vi "Main.vi"(11 "Module Admin":refnum<class "Delacor_lib_QMH_Module Admin.lvclass">) -> ()   [LabVIEW 2020, in "Interface Change.lvlib"]
doc: "This template is based off of the Queued Message Handler design pattern and the Queued Message Handler project template that ships with LabVIEW.\n\nThe main difference is that the queue is private to this module and communication between modules is performed via Broadcast and Request events.\n\nRequest events are wrapped in public API methods and are handled in the Event Handling Loop (EHL) of this VI. Any module can register for Broadcast events sent by this module. The EHL generates messages based on user interface actions.\n\nThe Message Handling Loop (MHL) processes messages generated by the EHL, or by other messages. The messages are string values, so new messages can be added easily to the Message Cases case structure in the MHL. Each message cluster can also provide an optional value for Message Data, which is a variant that can be converted to whatever message-specific data is required.\n_____\nBased on DQMH Project Template 6.1.0.94."
uses:
  Interface Change.lvlib
  <vilib>/Delacor/Delacor QMH/Libraries/Module Admin_class/Delacor_lib_QMH_Module Admin.lvclass
  Module Data--cluster.ctl
  <vilib>/Delacor/Delacor QMH/Libraries/Message Queue_class/Delacor_lib_QMH_Message Queue.lvclass/Delacor_lib_QMH_Message Queue.ctl
  Stop Argument--cluster.ctl
  <vilib>/Delacor/Delacor QMH/Libraries/Module Admin_class/Delacor_lib_QMH_Module Admin.lvclass/Delacor_lib_QMH_Module Admin.ctl
  Change ColorBox Argument--cluster.ctl
  <vilib>/Utility/miscctls.llb/LVPointTypeDef.ctl
  <vilib>/Delacor/Delacor QMH/Libraries/Message Queue_class/Delacor_lib_QMH_Enqueue Message (Single).vi
  <vilib>/Delacor/Delacor QMH/Libraries/Module Admin_class/Delacor_lib_QMH_Get External Launch.vi
  <vilib>/Utility/error.llb/Error Cluster From Error Code.vi
  <vilib>/ErrorRing/Error Ring.xnode
  <vilib>/Delacor/Delacor QMH/Libraries/Message Queue_class/Delacor_lib_QMH_Message Queue.lvclass
panel:
  out "error out":errorcluster
  in  "Simulate MHL Error":bool
  in  "Simulate EHL Error":bool
  # "Other QMH Modules communicate with this Module via its Public API (wrappers for its Request Events).\n\nThis Module communicates with other Modules via its Broadcast Events.\nAny module that wants to get these messages, just registers for this module's Broadcast events."
  # "This template is for the Delacor Modified Queued Message Handler design pattern.\n\nSee the block diagram for more information on how to use this template."
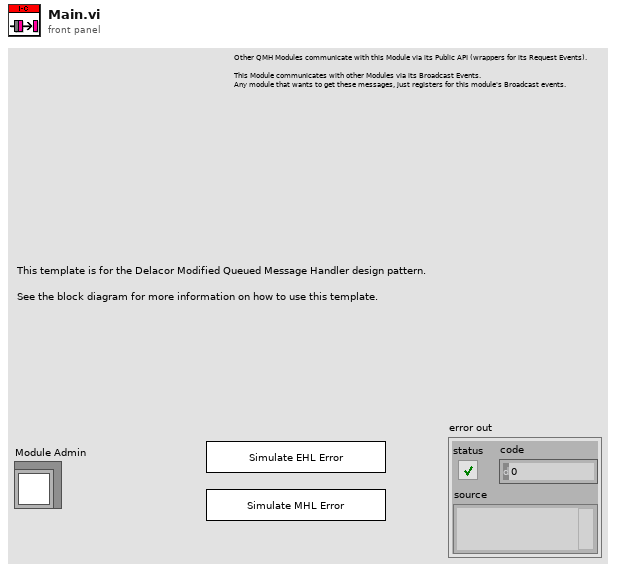
[diagram p1: front panel]
types:
  T1 = typedef "Interface Change.lvlib/Request Events--cluster.ctl" = cluster{"Stop Module":refnum<user-event>, "Show Panel":refnum<user-event>, "Hide Panel":refnum<user-event>, "Get Module Execution Status":refnum<user-event>, "Show Diagram":refnum<user-event>, "Change ColorBox":refnum<user-event>}
  T2 = typedef "Interface Change.lvlib/Module Data--cluster.ctl" = cluster{"Status":string}
  T3 = enum32{"invalid lock state", "Not Locked", "Locked (No Password)", "Password-protected"}
  T4 = typedef "Interface Change.lvlib/Stop Argument--cluster.ctl" = cluster{"Origin":string, "Exit via Stop Module Req?":bool, "Wait for Module to stop?":bool}
  T5 = typedef "Interface Change.lvlib/Change ColorBox Argument--cluster.ctl" = cluster{"Color Box":u32}
  T6 = typedef "LVPointTypeDef.ctl" = cluster{"Horizontal":i16, "Vertical":i16}
  T7 = enum32{"Invalid", "Standard", "Closed", "Hidden", "Minimized", "Maximized"}
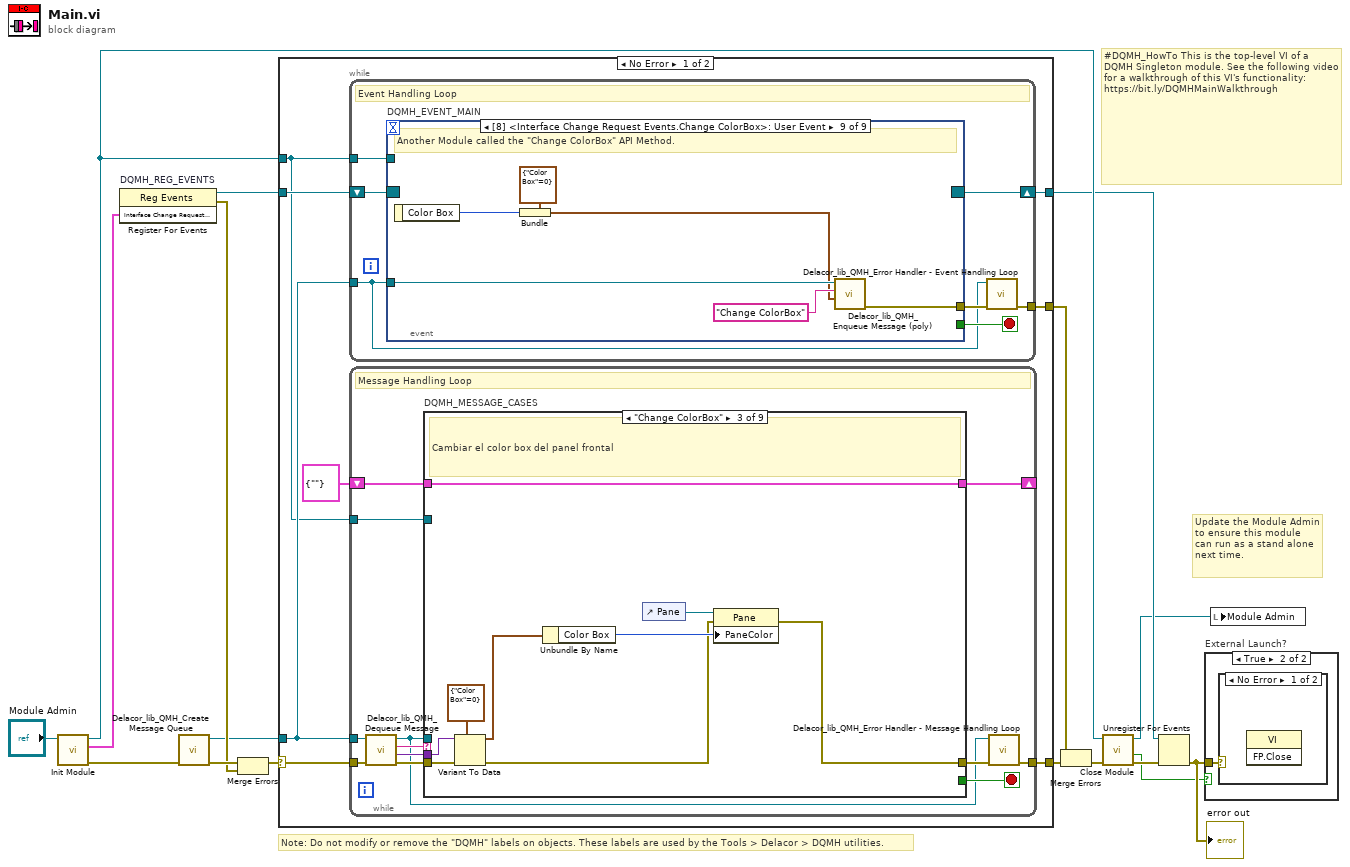
[diagram p0: block diagram]
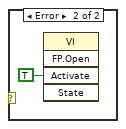
[diagram p3: hidden frame]
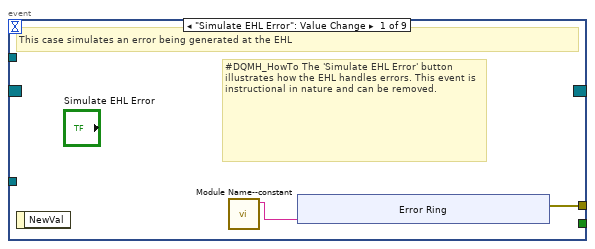
[diagram p4: hidden frame]
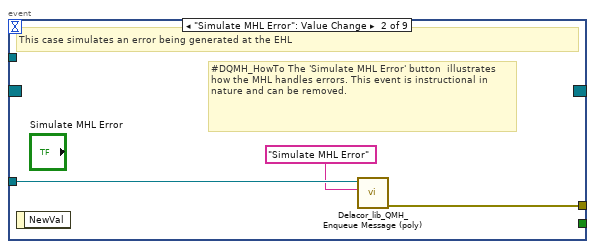
[diagram p5: hidden frame]
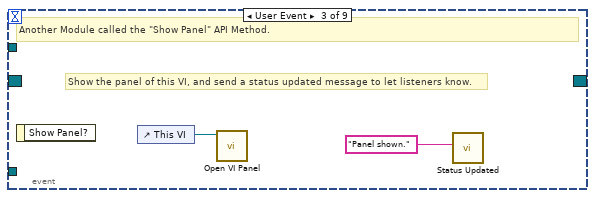
[diagram p6: hidden frame]
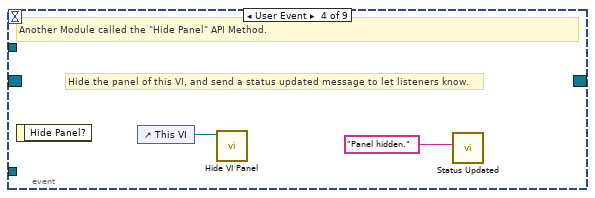
[diagram p7: hidden frame]
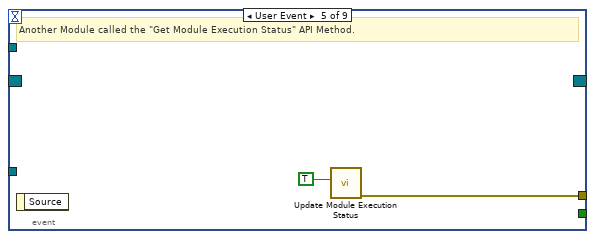
[diagram p8: hidden frame]
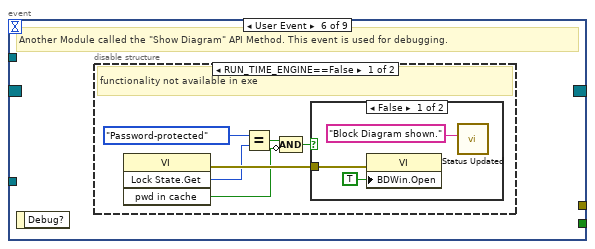
[diagram p9: hidden frame]
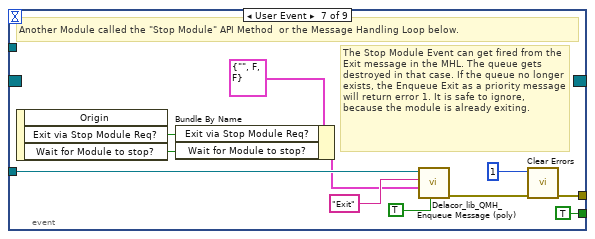
[diagram p12: hidden frame]
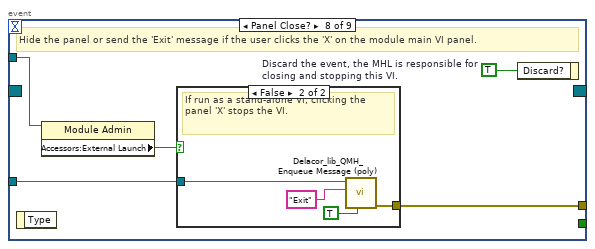
[diagram p13: hidden frame]
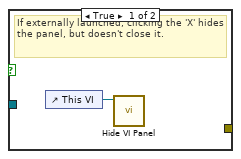
[diagram p14: hidden frame]
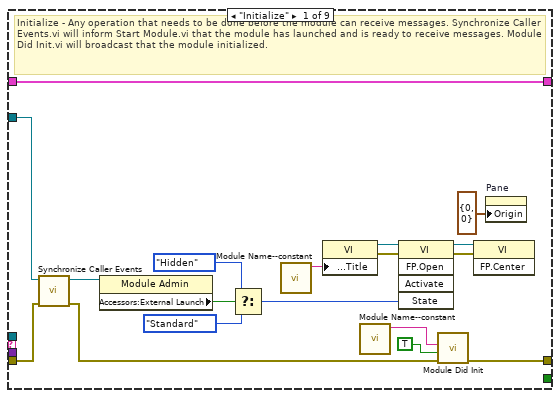
[diagram p15: hidden frame]
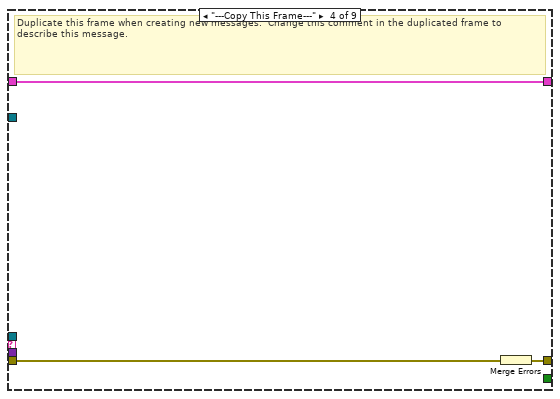
[diagram p17: hidden frame]
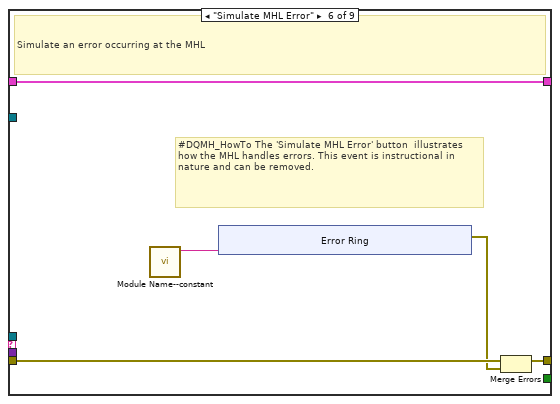
[diagram p19: hidden frame]
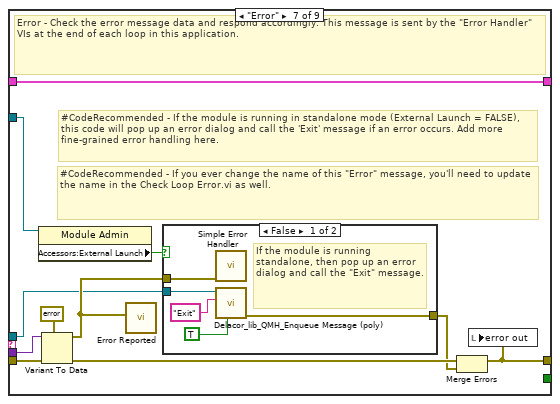
[diagram p20: hidden frame]
diagram:
  # "#DQMH_HowTo This is the top-level VI of a DQMH Singleton module. See the following video for a walkthrough of this VI's functionality: https://bit.ly/DQMHMainWalkthrough"
  # "Note: Do not modify or remove the \"DQMH\" labels on objects. These labels are used by the Tools > Delacor > DQMH utilities."
  # "Update the Module Admin to ensure this module can run as a stand alone next time."
  n1 = call "Init Module.vi"("Singleton Module Admin in"="Module Admin") -> ("error out"=w16:errorcluster, "Interface Change Request Events"=w5:T1, "Singleton Module Admin out"=w8:refnum<class "Delacor_lib_QMH_Module Admin.lvclass">)  [unwired: 8 in]
  n2 = register-events "DQMH_REG_EVENTS"(w5) -> (reference out=w6:refnum<event-registration>, error out=w9:errorcluster)  [unwired: 2 in]
  n3 = call <vilib>:"Delacor_lib_QMH_Create Message Queue.vi"("error in"=w16) -> ("error out"=w11:errorcluster, "Message Queue"=w4:refnum<class "Delacor_lib_QMH_Message Queue.lvclass">)  [unwired: 9 in]
  n4 = Merge Errors(w11, w9) -> (w10:errorcluster)
  n5 = case shown="No Error" w10 {
    selector: w10 -> [w23 w192]
    tunnel: [w25 w191] -> w17
    tunnel: [w22 w197] -> w7
    tunnel: w6 -> [w20 w197]
    tunnel: w4 -> [w19 w190]
    tunnel: [w24 _] -> w14
    tunnel: w8 -> [w18 w193]
    frame No Error {
      n6 = while {
        tunnel: w19 -> [w26]
        shift-right: [w29] -> w22
        shift-left: w20 -> [w30]
        tunnel: [w31] -> w24
        tunnel: w18 -> [w27]
        stop <- w28 stop-if-true
        # "Event Handling Loop"
        n7 = event "DQMH_EVENT_MAIN" shown="[8] <Interface Change Request Events.Change ColorBox>: User Event" {
          selector: w30 -> [_ _ _ _ _ _ _ _ _]
          dyn-events: [_ _ _ _ _ _ _ _ _] -> w29
          timeout: _ -> [_ _ _ _ _ _ _ _ _]
          tunnel: [_ _ _ _ _ _ TRUE ("Discard?") _ _] -> w28
          tunnel: w26 -> [_ w43 _ _ _ _ w66 w73 w86]
          tunnel: [w34 w44 _ _ w50 _ w69 w75 w81] -> w32
          tunnel: w27 -> [_ _ _ _ _ _ _ w72 _]
          event "Simulate EHL Error": Value Change {
            # "#DQMH_HowTo The 'Simulate EHL Error' button  illustrates how the EHL handles errors. This event is instructional in nature and can be removed."
            # "This case simulates an error being generated at the EHL"
            n8 = event-data() -> ()  [unwired: 1 in, 1 out]
            n9 = call "Module Name--constant.vi"() -> ("Module Name"=w33:string)  [unwired: 11 in]
            n10 = xnode "Error Ring"("parameter 0"=w33) -> ("error out"=w34:errorcluster)
          }
          event "Simulate MHL Error": Value Change {
            # "#DQMH_HowTo The 'Simulate MHL Error' button  illustrates how the MHL handles errors. This event is instructional in nature and can be removed."
            # "This case simulates an error being generated at the EHL"
            n11 = event-data() -> ()  [unwired: 1 in, 1 out]
            n12 = call-poly <vilib>:"Delacor_lib_QMH_Enqueue Message (poly).vi"("Message"="Simulate MHL Error", "Message Queue in"=w43) -> ("error out"=w44:errorcluster)  [unwired: 8 in, 1 out]
          }
          event User Event {
            # "Show the panel of this VI, and send a status updated message to let listeners know."
            # "Another Module called the \"Show Panel\" API Method."
            n13 = event-data() -> ()  [unwired: 1 in, 1 out]
            n14 = control-ref of="This VI"() -> (w46:refnum<vi>)
            n15 = call "Open VI Panel.vi"("VI"=w46) -> ()  [unwired: 10 in, 1 out]
            n16 = call "Status Updated.vi"("Status"="Panel shown." ("format string")) -> ()  [unwired: 10 in, 1 out]
          }
          event User Event {
            # "Hide the panel of this VI, and send a status updated message to let listeners know."
            # "Another Module called the \"Hide Panel\" API Method."
            n17 = event-data() -> ()  [unwired: 1 in, 1 out]
            n18 = control-ref of="This VI"() -> (w48:refnum<vi>)
            n19 = call "Hide VI Panel.vi"("VI"=w48) -> ()  [unwired: 10 in, 1 out]
            n20 = call "Status Updated.vi"("Status"="Panel hidden." ("format string")) -> ()  [unwired: 10 in, 1 out]
          }
          event User Event {
            # "Another Module called the \"Get Module Execution Status\" API Method."
            n21 = event-data() -> ()  [unwired: 1 in, 1 out]
            n22 = call "Update Module Execution Status.vi"("Running?"=TRUE) -> ("error out"=w50:errorcluster)  [unwired: 10 in]
          }
          event User Event {
            # "Another Module called the \"Show Diagram\" API Method. This event is used for debugging."
            n23 = event-data() -> ()  [unwired: 1 in, 1 out]
            n24 = disable-structure shown="RUN_TIME_ENGINE==False" {
              frame condition #0 (active) {
                # "functionality not available in exe"
                n25 = invoke class="VI" method="Lock State.Get"() -> (error out=w56:errorcluster, "Get Lock State"=w55:T3, "pwd in cache"=w52:bool)  [unwired: 4 in, 1 out]
                n26 = Equal?(x=T3."Password-protected", y=w55) -> (x = y?=w53:bool)
                n27 = Compound Arithmetic op=AND(w53, invert w52) -> (w51:bool)
                n28 = case shown="False" w51 {
                  tunnel: w56 -> [w59 _]
                  frame False {
                    n29 = property class="VI"(error in=w59, "BDWin.Open"=TRUE ("Block Diagram Window:Open")) -> ()  [unwired: 1 in, 2 out]
                    n30 = call "Status Updated.vi"("Status"="Block Diagram shown." ("format string")) -> ()  [unwired: 10 in, 1 out]
                  }
                  frame True {
                    # "Password-protected VI, and the password is not in the cache. Do not show the diagram."
                  }
                }
              }
              frame condition #1 {
              }
            }
          }
          event User Event {
            # "The Stop Module Event can get fired from the Exit message in the MHL. The queue gets destroyed in that case. If the queue no longer exists, the Enqueue Exit as a priority message will return error 1. It is safe to ignore, because the module is already exiting."
            # "Another Module called the \"Stop Module\" API Method  or the Message Handling Loop below."
            n31 = event-data() -> ("Exit via Stop Module Req?"=w62:bool, "Wait for Module to stop?"=w61:bool)  [unwired: 1 in, 1 out]
            n32 = Bundle By Name(cluster=T4 {"Origin"="", "Exit via Stop Module Req?"=FALSE, "Wait for Module to stop?"=FALSE} ("Stop Argument"), "Exit via Stop Module Req?"=w62, "Wait for Module to stop?"=w61) -> (w60:T4)
            n33 = call-poly <vilib>:"Delacor_lib_QMH_Enqueue Message (poly).vi"("Priority Message? (F)"=TRUE, "Message Data"=w60, "Message"="Exit", "Message Queue in"=w66) -> ("error out"=w70:errorcluster)  [unwired: 6 in, 1 out]
            n34 = call <vilib>:"Clear Errors.vi"("error in (no error)"=w70, "specific error code to clear (0: all)"=1) -> ("error out"=w69:errorcluster)  [unwired: 4 in, 1 out]
          }
          event Panel Close? {
            w74 = TRUE  # Discard the event, the MHL is responsible for closing and stopping this VI.
            # "Hide the panel or send the 'Exit' message if the user clicks the 'X' on the module main VI panel."
            n35 = event-data() -> ()  [unwired: 1 in, 1 out]
            n36 = property class="Module Admin"(reference=w72) -> ("Accessors:External Launch"=w71:bool)  [unwired: 1 in, 2 out]
            n37 = case shown="False" w71 {
              tunnel: w73 -> [_ w79]
              tunnel: [_ w80] -> w75
              frame True {
                # "If externally launched, clicking the 'X' hides the panel, but doesn't close it."
                n38 = control-ref of="This VI"() -> (w76:refnum<vi>)
                n39 = call "Hide VI Panel.vi"("VI"=w76) -> ()  [unwired: 10 in, 1 out]
              }
              frame False {
                # "If run as a stand-alone VI, clicking the panel 'X' stops the VI."
                n40 = call-poly <vilib>:"Delacor_lib_QMH_Enqueue Message (poly).vi"("Priority Message? (F)"=TRUE, "Message"="Exit", "Message Queue in"=w79) -> ("error out"=w80:errorcluster)  [unwired: 7 in, 1 out]
              }
            }
            n41 = event-data("Discard?"=w74) -> ()  [unwired: 1 in, 1 out]
          }
          event User Event {
            # "Another Module called the \"Change ColorBox\" API Method."
            n42 = event-data() -> ("Color Box"=w82:u32)  [unwired: 1 in]
            n43 = Bundle(cluster=T5 {"Color Box"=0} ("Change ColorBox Argument"), "Color Box"=w82) -> (w83:T5)
            n44 = call-poly <vilib>:"Delacor_lib_QMH_Enqueue Message (poly).vi"("Message Data"=w83, "Message"="Change ColorBox", "Message Queue in"=w86) -> ("error out"=w81:errorcluster)  [unwired: 7 in, 1 out]
          }
        }
        n45 = call-dynamic "Delacor_lib_QMH_Error Handler - Event Handling Loop.vi"("error in"=w32, "Message Queue in"=w26) -> ("dup error in"=w31:errorcluster)  [unwired: 8 in, 1 out]
      }
      n46 = while {
        tunnel: w19 -> [w89]
        shift-right: [w93] -> _
        shift-left: T2 {"Status"=""} ("Data Cluster") -> [w94]
        tunnel: w23 -> [w97]
        tunnel: [w95] -> w25
        tunnel: w18 -> [w87]
        stop <- w92 stop-if-true
        # "Message Handling Loop"
        n47 = call-dynamic "Delacor_lib_QMH_Dequeue Message.vi"("error in"=w97, "Message Queue in"=w89) -> ("error out"=w96:errorcluster, "Message Data"=w90:variant, "Message"=w91:string, "Message Queue out"=w88:refnum<class "Delacor_lib_QMH_Message Queue.lvclass">)  [unwired: 6 in]
        n48 = case "DQMH_MESSAGE_CASES" shown="\"Change ColorBox\"" w91 {
          selector: w91 -> [_ _ _ _ _ _ _ _ w177]
          tunnel: w88 -> [_ _ _ _ _ _ w147 w169 _]
          tunnel: w96 -> [w114 w118 w127 w130 w132 w137 w154 w175 w179]
          tunnel: [w112 w118 w119 w129 w132 w136 w150 w172 w180] -> w98
          tunnel: w94 -> [w99 w117 w126 w128 w131 w134 w149 w168 w178]
          tunnel: [w99 w117 w126 w128 w131 w134 w149 w168 w178] -> w93
          tunnel: [_ _ _ _ _ _ _ w167 _] -> w92
          tunnel: w90 -> [_ _ w125 _ _ _ w148 w166 _]
          tunnel: w87 -> [w104 _ _ _ _ _ w146 w161 _]
          frame "Initialize" {
            # "Initialize - Any operation that needs to be done before the module can receive messages. Synchronize Caller Events.vi will inform Start Module.vi that the module has launched and is ready to receive messages. Module Did Init.vi will broadcast that the module initialized."
            n49 = call "Synchronize Caller Events.vi"("error in (no error)"=w114, "Singleton Module Admin in"=w104) -> ("error out"=w113:errorcluster, "Singleton Module Admin out"=w101:refnum<class "Delacor_lib_QMH_Module Admin.lvclass">)  [unwired: 8 in]
            n50 = property class="Module Admin"(reference=w101) -> ("Accessors:External Launch"=w108:bool)  [unwired: 1 in, 2 out]
            n51 = Select(t=T7."Hidden" ("State"), s=w108, f=T7."Standard" ("State")) -> (s? t:f=w105:T7)
            n52 = call "Module Name--constant.vi"() -> ("Module Name"=w111:string)  [unwired: 11 in]
            n53 = property class="VI"("Front Panel.Title"=w111) -> (reference out=w110:refnum<vi>, error out=w116:errorcluster)  [unwired: 2 in]
            n54 = call "Module Name--constant.vi"() -> ("Module Name"=w102:string)  [unwired: 11 in]
            n55 = invoke class="VI" method="FP.Open"(reference=w110, error in=w116, "State"=w105) -> (reference out=w109:refnum<vi>, error out=w115:errorcluster)  [unwired: 2 in, 3 out]
            n56 = call "Module Did Init.vi"("error in (no error)"=w113, "Initialized?"=TRUE, "Origin"=w102) -> ("error out"=w112:errorcluster)  [unwired: 8 in]
            n57 = invoke class="VI" method="FP.Center"(reference=w109, error in=w115) -> ()  [unwired: 1 in, 3 out]
            n58 = property on="Pane" class="Pane"("Origin"=T6 {"Horizontal"=0, "Vertical"=0}) -> ()  [unwired: 2 in, 2 out]
          }
          frame "---Module Specific---" {
            # "Separator -- The following cases handle messages specific to this Module."
          }
          frame "Change ColorBox" {
            # "Cambiar el color box del panel frontal"
            n59 = Variant To Data(error in=w127, type=T5 {"Color Box"=0} ("Change ColorBox Argument"), Variant=w125) -> (data=w123:T5, error out=w120:errorcluster)
            n60 = Unbundle By Name(w123) -> ("Color Box"=w121:u32)
            n61 = control-ref of="Pane"() -> (w122:refnum<vi>)
            n62 = property class="Pane"(reference=w122, error in=w120, "PaneColor"=w121) -> (error out=w119:errorcluster)  [unwired: 1 out]
          }
          frame "---Copy This Frame---" {
            # "Duplicate this frame when creating new messages.  Change this comment in the duplicated frame to describe this message."
            n63 = Merge Errors(w130) -> (w129:errorcluster)
          }
          frame "---Exit and Error Handling---" {
            # "Separator - The following cases handle errors and exit messages."
          }
          frame "Simulate MHL Error" {
            # "#DQMH_HowTo The 'Simulate MHL Error' button  illustrates how the MHL handles errors. This event is instructional in nature and can be removed."
            # "Simulate an error occurring at the MHL"
            n64 = call "Module Name--constant.vi"() -> ("Module Name"=w133:string)  [unwired: 11 in]
            n65 = xnode "Error Ring"("parameter 0"=w133) -> ("error out"=w135:errorcluster)
            n66 = Merge Errors(w137, w135) -> (w136:errorcluster)
          }
          frame "Error" {
            # "#CodeRecommended - If you ever change the name of this \"Error\" message, you'll need to update the name in the Check Loop Error.vi as well."
            # "#CodeRecommended - If the module is running in standalone mode (External Launch = FALSE), this code will pop up an error dialog and call the 'Exit' message if an error occurs. Add more fine-grained error handling here."
            # "Error - Check the error message data and respond accordingly. This message is sent by the \"Error Handler\" VIs at the end of each loop in this application."
            n67 = property class="Module Admin"(reference=w146) -> ("Accessors:External Launch"=w145:bool)  [unwired: 1 in, 2 out]
            n68 = Variant To Data(error in=w154, type=errorcluster {"status"=FALSE, "code"=0, "source"=""} ("error constant"), Variant=w148) -> (data=w155:errorcluster, error out=w152:errorcluster)
            n69 = call "Error Reported.vi"("Error"=w155) -> ()  [unwired: 10 in, 1 out]
            n70 = case shown="False" w145 {
              tunnel: [w160 _] -> w151
              tunnel: w147 -> [w158 _]
              tunnel: w155 -> [w159 _]
              frame False {
                # "If the module is running standalone, then pop up an error dialog and call the \"Exit\" message."
                n71 = call <vilib>:"Simple Error Handler.vi"("error in (no error)"=w159) -> ()  [unwired: 4 in, 5 out]
                n72 = call-poly <vilib>:"Delacor_lib_QMH_Enqueue Message (poly).vi"("Priority Message? (F)"=TRUE, "Message"="Exit", "Message Queue in"=w158) -> ("error out"=w160:errorcluster)  [unwired: 7 in, 1 out]
              }
              frame True {
                # "If the module was launched externally, calling the Error Reported broadcast VI is the only action performed by the \"Error\" message. The module's caller can then process the error appropriately."
              }
            }
            n73 = Merge Errors(w152, w151) -> (w150:errorcluster)
            n74 = local write "error out"(w150) -> ()
          }
          frame "Exit" {
            w165 = 91  # 91: not all Exit messages will have an argument
            w167 = TRUE  # Stop the VI
            # "Release the message queue reference"
            # "#CodeNeeded - Add any required cleanup code here"
            # "Exit - Exit the application."
            n75 = Variant To Data(error in=w175, type=T4 {"Origin"="", "Exit via Stop Module Req?"=FALSE, "Wait for Module to stop?"=FALSE} ("Stop Argument"), Variant=w166) -> (data=w163:T4, error out=w171:errorcluster)
            n76 = call <vilib>:"Clear Errors.vi"("error in (no error)"=w171, "specific error code to clear (0: all)"=w165) -> ("error out"=w174:errorcluster)  [unwired: 4 in, 1 out]
            n77 = control-ref of="This VI"() -> (w162:refnum<vi>)
            n78 = call-dynamic "Delacor_lib_QMH_Release Message Queue.vi"("error in"=w174, "Message Queue"=w169) -> ("error out"=w173:errorcluster)  [unwired: 9 in]
            n79 = call "Handle Exit.vi"("Stop Argument"=w163, "Admin in"=w161, "VI reference"=w162) -> ("error out"=w170:errorcluster)  [unwired: 7 in, 1 out]
            n80 = Merge Errors(w173, w170) -> (w172:errorcluster)
          }
          frame Default {
            # "'Default' case only runs if there is a message that isn't defined in any of the other cases.  Output a programming error."
            n81 = call "Module Name--constant.vi"() -> ("Module Name"=w176:string)  [unwired: 11 in]
            n82 = xnode "Error Ring"("parameter 0"=w177, "parameter 1"=w176) -> ("error out"=w181:errorcluster)
            n83 = Merge Errors(w179, w181) -> (w180:errorcluster)
          }
        }
        n84 = call-dynamic "Delacor_lib_QMH_Error Handler - Message Handling Loop.vi"("error in"=w98, "Message Queue in"=w88) -> ("dup error in"=w95:errorcluster)  [unwired: 8 in, 1 out]
      }
    }
    frame Error {
      # "Synchronize Caller Events.vi will inform Start Module.vi that the module has launched and will let the code calling Start Module.vi register for broadcasts and would permit the caller receive the broadcast that an error occurred at launch time."
      n85 = call-dynamic "Delacor_lib_QMH_Release Message Queue.vi"("error in"=w192, "Message Queue"=w190) -> ("error out"=w191:errorcluster)  [unwired: 9 in]
      n86 = call "Synchronize Caller Events.vi"("Singleton Module Admin in"=w193) -> ("error out"=w198:errorcluster)  [unwired: 9 in, 1 out]
      n87 = call "Module Name--constant.vi"() -> ("Module Name"=w196:string)  [unwired: 11 in]
      n88 = Format Into String(format string="An error occurred during initialization. %s is no longer running.", w196) -> (resulting string=w194:string)  [unwired: 2 in, 1 out]
      n89 = Merge Errors(w191, w198) -> (w199:errorcluster)
      n90 = call "Error Reported.vi"("Additional Information"=w194, "Error"=w199) -> ()  [unwired: 9 in, 1 out]
    }
  }
  n91 = Merge Errors(w14, w17) -> (w13:errorcluster)
  n92 = call "Close Module.vi"("error in (no error)"=w13, "Module Admin in"=w8) -> ("error out"=w15:errorcluster, "External Launch"=w1:bool, "Module Admin out"=w2:refnum<class "Delacor_lib_QMH_Module Admin.lvclass">)  [unwired: 7 in]
  n93 = Unregister For Events(event registration refnum=w7, error in=w15) -> (error out=w12:errorcluster)
  "error out" <- w12
  n94 = case "External Launch?" shown="True" w1 {
    tunnel: w12 -> [_ w200]
    frame False {
    }
    frame True {
      n95 = case shown="No Error" w200 {
        frame No Error {
          n96 = invoke class="VI" method="FP.Close"() -> ()  [unwired: 3 in, 3 out]
        }
        frame Error {
          n97 = invoke class="VI" method="FP.Open"("Activate"=TRUE ("Activate?")) -> ()  [unwired: 4 in, 5 out]
        }
      }
    }
  }
  n98 = local write "Module Admin"(w2) -> ()
